vi "Parse Path.vi"(8 "error in":errorcluster, 11 "Path String":string) -> (0 "error out":errorcluster, 3 "Path":cluster{"ID / Name":variant, "Index":i32}[](array[cluster]))   [LabVIEW 2020, in "Protobuf RAW.lvlib" / "Raw Message.lvclass"]
uses:
  Raw Message.lvclass
  <vilib>/regexp/Match Regular Expression.xnode
  Raw Message.lvclass/Raw Message.ctl
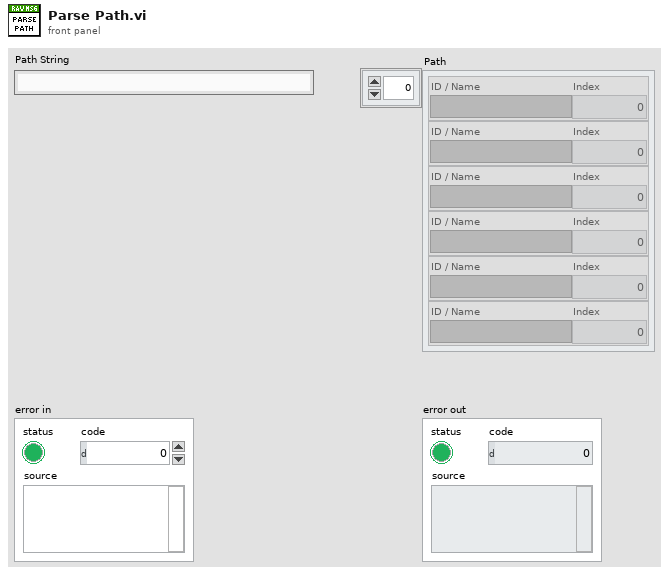
[diagram p1: front panel]
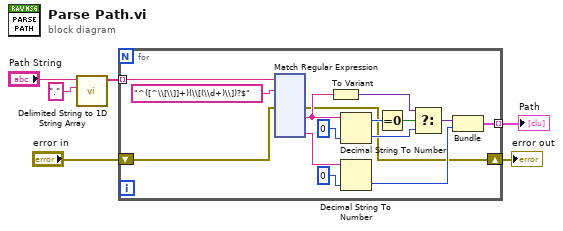
[diagram p0: block diagram]
diagram:
  n1 = call <vilib>:"Delimited String to 1D String Array.vi"("delimiter"=".", "delimited string"="Path String") -> ("string array"=w4:string[])  [unwired: 9 in]
  n2 = for {
    tunnel: w4 -> [w16] mode=indexing
    tunnel: [w10] -> w3 mode=indexing
    shift-right: [w7] -> w1
    shift-left: "error in" -> [w8]
    n3 = xnode "Match Regular Expression"("input string"=w16, "regular expression"="^([^\\[\\]]+)(\\[(\\d+)\\])?$", "error in"=w8) -> ("error out"=w7:errorcluster, "submatch 1"=w14:string, "submatch 3"=w9:string)  [unwired: 3 in, 5 out]
    n4 = To Variant(anything=w14) -> (Variant=w18:variant)
    n5 = Decimal String To Number(string=w14, default (0L)=u32 0 ("default (0 I32)")) -> (offset past number=w20:i32, number=w17:u32)  [unwired: 1 in]
    n6 = Decimal String To Number(string=w9, default (0L)=0 ("default (0 I32)")) -> (number=w11:i32)  [unwired: 1 in, 1 out]
    n7 = Equal To 0?(x=w20) -> (x = 0?=w19:bool)
    n8 = Select(t=w18, s=w19, f=w17) -> (s? t:f=w12:variant)
    n9 = Bundle("Variant"=w12, w11) -> (w10:cluster{"Variant":variant, i32})  [unwired: 1 in]
  }
  "Path" <- w3
  "error out" <- w1
